vi "Motor_Begin.vi"   [LabVIEW 2015]
uses:
  <vilib>/Rock Robotics/WPI/SafetyOutput/WPI_SafetyOutputConfigMenu.ctl
  <vilib>/Rock Robotics/WPI/CAN/TalonSRX/WPI_CANTalonSRX_APIControlMode.ctl
  Global_Var/Drive_Global.vi
  <vilib>/Rock Robotics/WPI/MotorControl/WPI_MotorControlOpenCANTalonSRX.vi
types:
  T1 = typedef "WPI_SafetyOutputConfigMenu.ctl" = enum16{"Enable", "Disable"}
  T2 = typedef "WPI_CANTalonSRX_APIControlMode.ctl" = enum8{"Percent VBus", "Speed", "Position", "Slave", "Unchanged / Invalid", "Voltage Compensation", "Current", "Motion Profile"}
  T3 = typedef "WPI_RobotDriveDevRef.ctl" = cluster{"DevStatus":errorcluster, "Motors[]":T4[], "Square Inputs":bool, "Max Output":dbl}
  T4 = typedef "WPI_MotorControlDeviceRef.ctl" = cluster{"DeviceStatus":errorcluster, "Type":T5, "PWM":cluster{"PWM Channel":T6, "DeadBand":T7}, "CAN":cluster{"Device Number":u8, "Control Mode":T8, "Semaphore":T9, "Max Vout":dbl, "TalonSRX Control Mode":T2}, "Invert":bool}
  T5 = typedef "WPI_MotorControlType.ctl" = enum16{"PWM", "CAN", "CANTalonSRX"}
  T6 = typedef "FPGA_DIOPWMChannel.ctl" = enum8{"PWM 0", "PWM 1", "PWM 2", "PWM 3", "PWM 4", "PWM 5", "PWM 6", "PWM 7", "PWM 8", "PWM 9", "PWM MXP 0", "PWM MXP 1", "PWM MXP 2", "PWM MXP 3", "PWM MXP 4", "PWM MXP 5", "PWM MXP 6", "PWM MXP 7", "PWM MXP 8", "PWM MXP 9", "Invalid"}
  T7 = typedef "WPI_PWMDeadband.ctl" = cluster{"Name":string, "maxPositivePwm":i32, "minPositivePwm":i32, "centerPwm":i32, "maxNegativePwm":i32, "minNegativePwm":i32, "angularRange":u16}
  T8 = typedef "WPI_CANJaguar_ControlMode.ctl" = enum8{"Percent VBus", "Current", "Speed", "Position", "Voltage"}
  T9 = typedef "Semaphore RefNum" = refnum<k1>
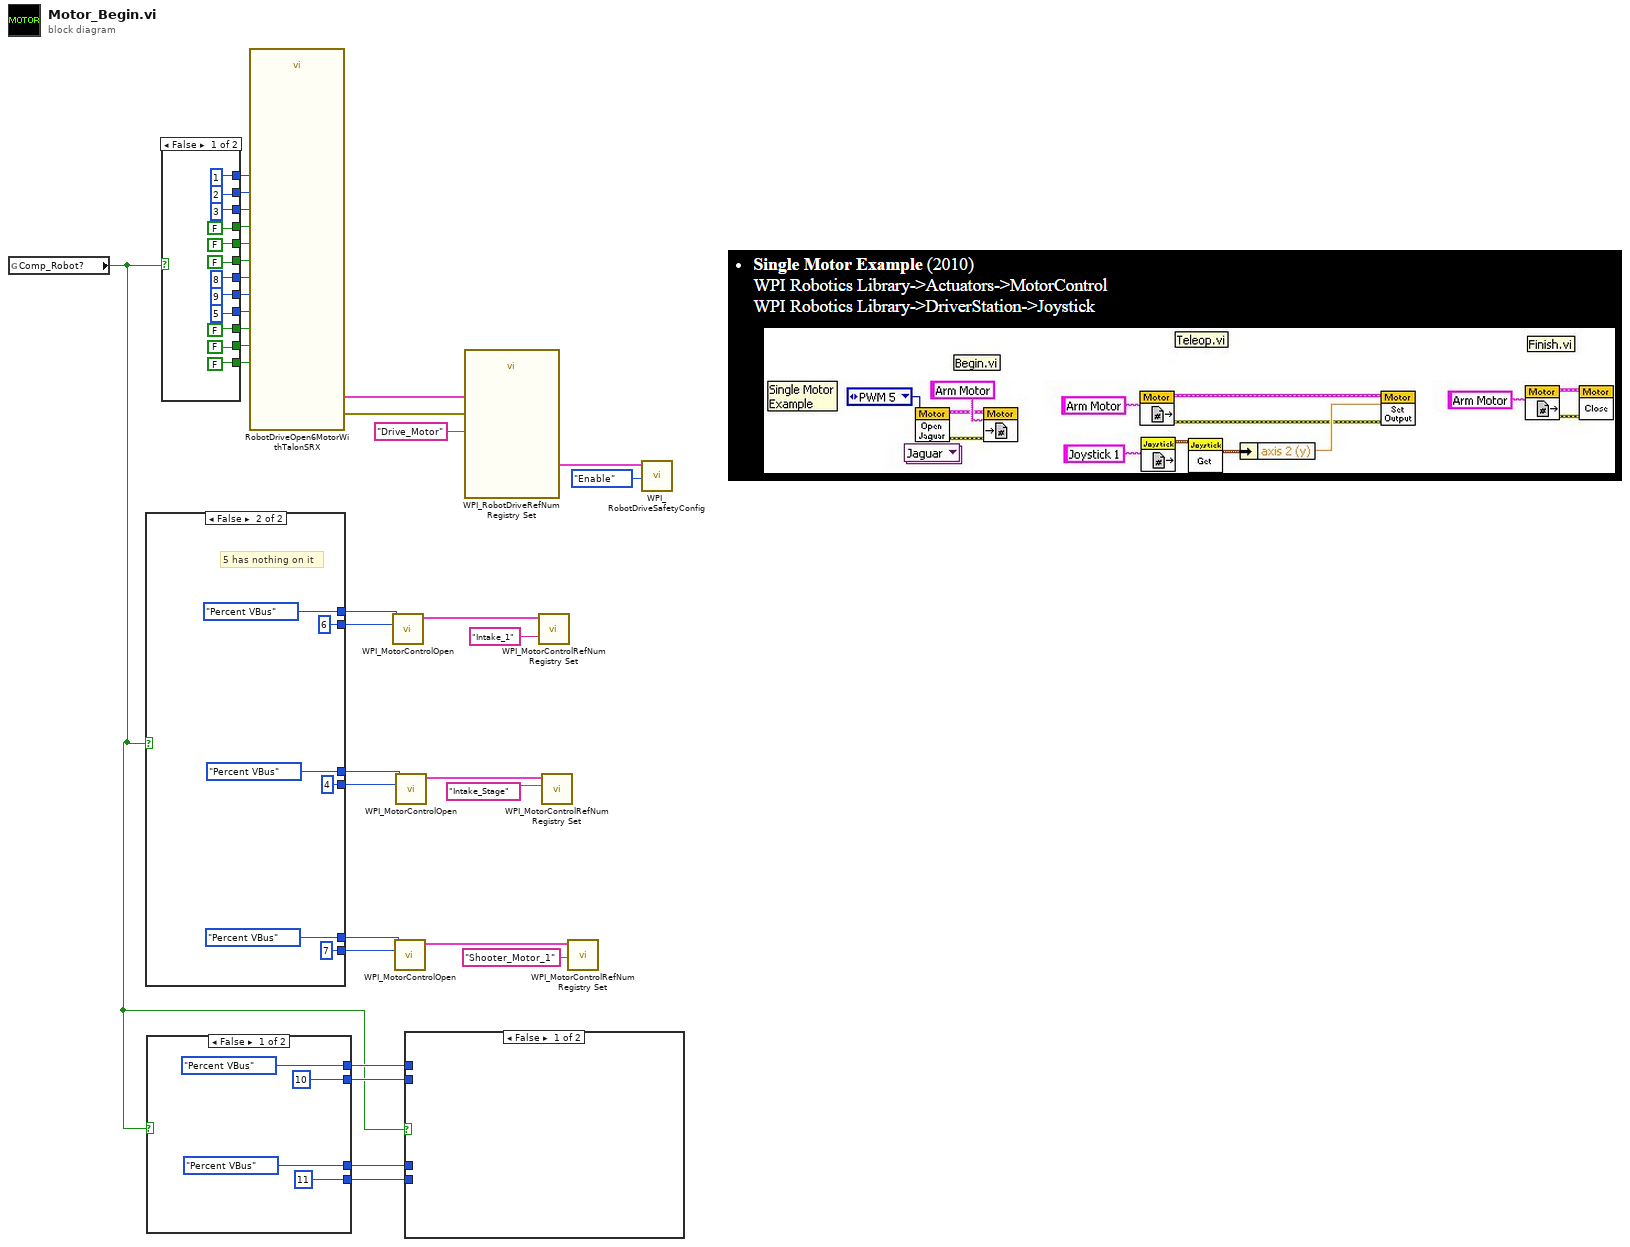
[diagram p0: block diagram]
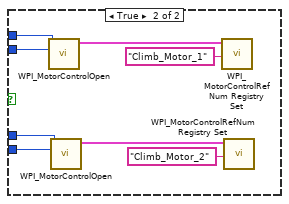
[diagram p2: hidden frame]
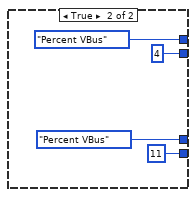
[diagram p3: hidden frame]
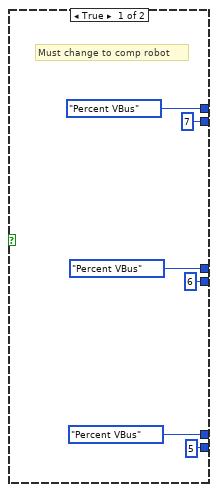
[diagram p4: hidden frame]
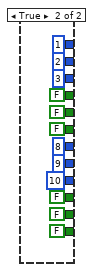
[diagram p5: hidden frame]
diagram:
  n1 = global read "Drive_Global.vi" "Comp_Robot?"() -> (w1:bool)
  n2 = case shown="False" w1 {
    tunnel: [WPI_CANTalonSRX_APIControlMode."Percent VBus" ("Control Mode") WPI_CANTalonSRX_APIControlMode."Percent VBus" ("Control Mode")] -> w16
    tunnel: [u8 7 ("Device Number") u8 6 ("Device Number")] -> w15
    tunnel: [WPI_CANTalonSRX_APIControlMode."Percent VBus" ("Control Mode") WPI_CANTalonSRX_APIControlMode."Percent VBus" ("Control Mode")] -> w13
    tunnel: [u8 6 ("Device Number") u8 4 ("Device Number")] -> w12
    tunnel: [WPI_CANTalonSRX_APIControlMode."Percent VBus" ("Control Mode") WPI_CANTalonSRX_APIControlMode."Percent VBus" ("Control Mode")] -> w10
    tunnel: [u8 5 ("Device Number") u8 7 ("Device Number")] -> w9
    frame True {
      # "Must change to comp robot"
    }
    frame False {
      # "5 has nothing on it"
    }
  }
  n3 = case shown="False" w1 {
    tunnel: [WPI_CANTalonSRX_APIControlMode."Percent VBus" ("Control Mode") WPI_CANTalonSRX_APIControlMode."Percent VBus" ("Control Mode")] -> w5
    tunnel: [u8 10 ("Device Number") u8 4 ("Device Number")] -> w4
    tunnel: [u8 11 ("Device Number") u8 11 ("Device Number")] -> w3
    tunnel: [WPI_CANTalonSRX_APIControlMode."Percent VBus" ("Control Mode") WPI_CANTalonSRX_APIControlMode."Percent VBus" ("Control Mode")] -> w2
    frame False {
    }
    frame True {
    }
  }
  n4 = case shown="False" w1 {
    tunnel: [u8 1 ("Left Motor 1") u8 1 ("Left Motor 1")] -> w30
    tunnel: [u8 2 ("Left Motor 2") u8 2 ("Left Motor 2")] -> w29
    tunnel: [u8 3 ("Left Motor 3") u8 3 ("Left Motor 3")] -> w28
    tunnel: [FALSE ("Left Motor Inverted 1") FALSE ("Left Motor Inverted 1")] -> w27
    tunnel: [FALSE ("Left Motor Inverted 2") FALSE ("Left Motor Inverted 2")] -> w26
    tunnel: [FALSE ("Left Motor Inverted 3") FALSE ("Left Motor Inverted 3")] -> w25
    tunnel: [u8 8 ("Right Motor 1") u8 8 ("Right Motor 1")] -> w24
    tunnel: [u8 9 ("Right Motor 2") u8 9 ("Right Motor 2")] -> w23
    tunnel: [u8 5 ("Right Motor 3") u8 10 ("Right Motor 3")] -> w22
    tunnel: [FALSE ("Right Motor Inverted 1") FALSE ("Right Motor Inverted 1")] -> w21
    tunnel: [FALSE ("Right Motor Inverted 2") FALSE ("Right Motor Inverted 2")] -> w20
    tunnel: [FALSE ("Right Motor Inverted 3") FALSE ("Right Motor Inverted 3")] -> w19
    frame False {
    }
    frame True {
    }
  }
  n5 = call "RobotDriveOpen6MotorWithTalonSRX.vi"("Left Motor 1"=w30, "Left Motor 2"=w29, "Left Motor 3"=w28, "Right Motor 1"=w24, "Right Motor 2"=w23, "Right Motor 3"=w22, "Left Motor Inverted 1"=w27, "Right Motor Inverted 1"=w21, "Left Motor Inverted 2"=w26, "Right Motor Inverted 2"=w20, "Left Motor Inverted 3"=w25, "Right Motor Inverted 3"=w19) -> ("RobotDriveDevRef"=w32:T3, "error out"=w31:errorcluster)  [unwired: 14 in]
  n6 = call-poly <vilib>:"WPI_MotorControlOpen.vi"("Device Number"=w15, "Control Mode"=w16) -> ("MotorControlDeviceRef"=w17:T4)  [unwired: 8 in, 1 out]
  n7 = call-poly <vilib>:"WPI_MotorControlOpen.vi"("Device Number"=w9, "Control Mode"=w10) -> ("MotorControlDeviceRef"=w11:T4)  [unwired: 8 in, 1 out]
  n8 = call-poly <vilib>:"WPI_MotorControlOpen.vi"("Device Number"=w12, "Control Mode"=w13) -> ("MotorControlDeviceRef"=w14:T4)  [unwired: 8 in, 1 out]
  n9 = case shown="False" w1 {
    tunnel: w5 -> [_ w84]
    tunnel: w4 -> [_ w83]
    tunnel: w3 -> [_ w82]
    tunnel: w2 -> [_ w81]
    frame False {
    }
    frame True {
      n10 = call-poly <vilib>:"WPI_MotorControlOpen.vi"("Device Number"=w83, "Control Mode"=w84) -> ("MotorControlDeviceRef"=w85:T4)  [unwired: 8 in, 1 out]
      n11 = call-poly <vilib>:"WPI_MotorControlOpen.vi"("Device Number"=w82, "Control Mode"=w81) -> ("MotorControlDeviceRef"=w80:T4)  [unwired: 8 in, 1 out]
      n12 = call <vilib>:"WPI_MotorControlRefNum Registry Set.vi"("refnum name"="Climb_Motor_1", "MotorControlDevRef"=w85) -> ()  [unwired: 8 in, 2 out]
      n13 = call <vilib>:"WPI_MotorControlRefNum Registry Set.vi"("refnum name"="Climb_Motor_2", "MotorControlDevRef"=w80) -> ()  [unwired: 8 in, 2 out]
    }
  }
  n14 = call <vilib>:"WPI_RobotDriveRefNum Registry Set.vi"("error in (no error)"=w31, "refnum name"="Drive_Motor", "RobotDriveDevRef"=w32) -> ("RobotDriveDevRef"=w33:T3)  [unwired: 1 in, 7 out]
  n15 = call <vilib>:"WPI_MotorControlRefNum Registry Set.vi"("refnum name"="Intake_1", "MotorControlDevRef"=w17) -> ()  [unwired: 8 in, 2 out]
  n16 = call <vilib>:"WPI_MotorControlRefNum Registry Set.vi"("refnum name"="Intake_Stage" ("Intake_2"), "MotorControlDevRef"=w14) -> ()  [unwired: 8 in, 2 out]
  n17 = call <vilib>:"WPI_MotorControlRefNum Registry Set.vi"("refnum name"="Shooter_Motor_1", "MotorControlDevRef"=w11) -> ()  [unwired: 8 in, 2 out]
  n18 = call <vilib>:"WPI_RobotDriveSafetyConfig.vi"("mode"=WPI_SafetyOutputConfigMenu."Enable", "RobotDriveDevRef"=w33) -> ()  [unwired: 8 in, 2 out]
